vi "game_top_VI.vi"() -> ()   [LabVIEW 2014]
uses:
  <vilib>/Utility/miscctls.llb/LVPositionTypeDef.ctl
panel:
  in  "Stage Effects:":T1={"bar description"="ball will  speed up when pass aera: ", "brick discription"="ball will teleport \nand change speed: ", "y speed up"="◆□◆□◆□", "In : "=16711680, "Out : "=16711680, "x speed up"="■\n△\n■\n△\n△"}
  in  "leave":bool
  in  "Note":string="Score is calculated by :\n1. number of bricks breaked\n2. clear time of each level"
  in  "into pos 2":T2={"Left"=288, "Top"=-12}
  in  "into Pos":T2={"Left"=623, "Top"=-12}
  in  "OK Button":bool
  in  "Introoductions :":T3={"Bar : "=100, "bar description"="Move bar with key: \n  △    ■    ◆    □", "brick discription"="Use the ball to\nbreak the bricks", "Brick : "=0, "Ball : "=TRUE} {"Bar :" scale=0.0..100.0}
  in  "title":string="Brick Breaking Game"
  out "Top Ten High Score":T4(array[cluster])=[{"Placing"=1.0, "Name"="", "Score"=0.0, "Date"=""}, {"Placing"=2.0, "Name"="", "Score"=0.0, "Date"=""}, {"Placing"=3.0, "Name"="", "Score"=0.0, "Date"=""}, {"Placing"=4.0, "Name"="", "Score"=0.0, "Date"=""}, {"Placing"=5.0, "Name"="", "Score"=0.0, "Date"=""}, {"Placing"=6.0, "Name"="", "Score"=0.0, "Date"=""}, {"Placing"=7.0, "Name"="", "Score"=0.0, "Date"=""}, {"Placing"=8.0, "Name"="", "Score"=0.0, "Date"=""}, {"Placing"=9.0, "Name"="", "Score"=0.0, "Date"=""}, {"Placing"=10.0, "Name"="", "Score"=0.0, "Date"=""}]
  in  "Your Score":i32
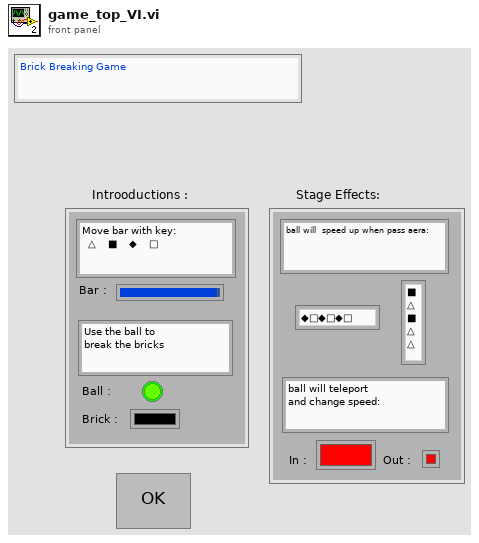
[diagram p1: front panel]
types:
  T1 = cluster{"bar description":string, "brick discription":string, "y speed up":string, "In : ":u32, "Out : ":u32, "x speed up":string}
  T2 = typedef "LVPositionTypeDef.ctl" = cluster{"Left":i32, "Top":i32}
  T3 = cluster{"Bar : ":u8, "bar description":string, "brick discription":string, "Brick : ":u32, "Ball : ":bool}
  T4 = cluster{"Placing":dbl, "Name":string, "Score":dbl, "Date":string}[]
  T5 = enum8{"Enabled", "Disabled", "Disabled and Grayed Out"}
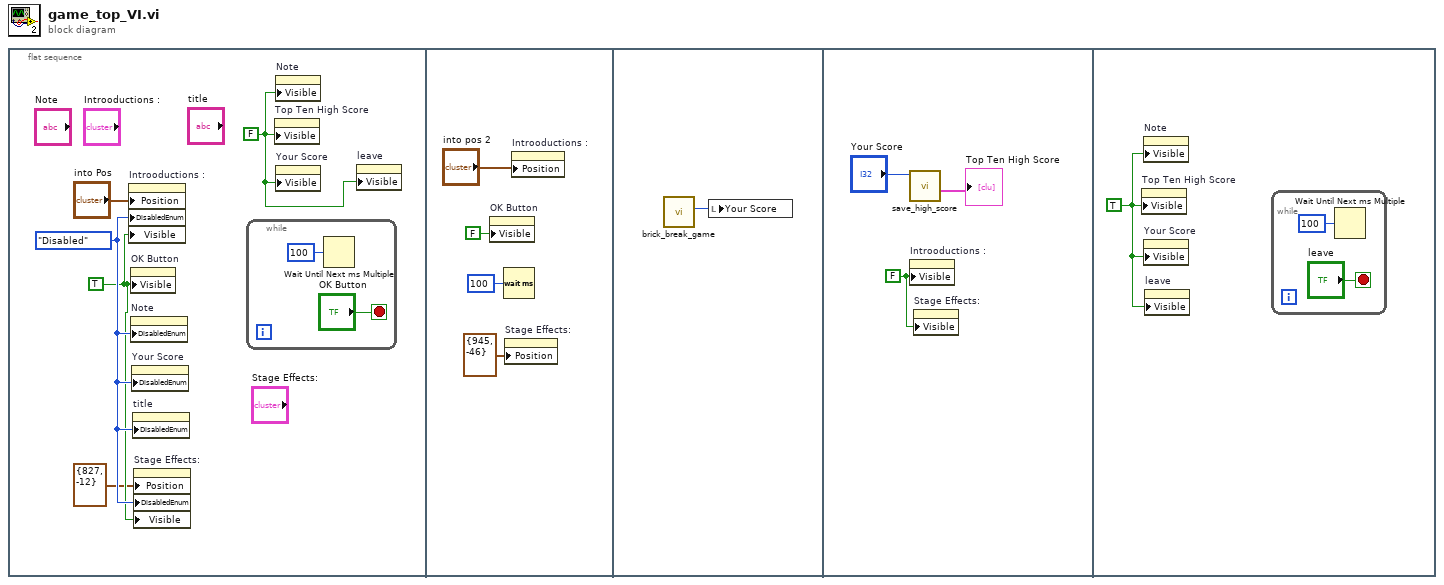
[diagram p0: block diagram]
diagram:
  n1 = flat-sequence {
    frame #0 {
      w4 = T5."Disabled" ("Disabled")
      w3 = TRUE ("Visible")
      w5 = FALSE
      n2 = property on="Introoductions :" class="Clust (strict)"("Position"="into Pos", "DisabledEnum"=w4, "Visible"=w3) -> ()  [unwired: 2 in, 2 out]
      n3 = property on="OK Button" class="Bool"("Visible"=w3) -> ()  [unwired: 2 in, 2 out]
      n4 = property on="Note" class="Str"("DisabledEnum"=w4) -> ()  [unwired: 2 in, 2 out]
      n5 = property on="Your Score" class="DigNum (strict)"("DisabledEnum"=w4) -> ()  [unwired: 2 in, 2 out]
      n6 = property on="title" class="Str"("DisabledEnum"=w4) -> ()  [unwired: 2 in, 2 out]
      n7 = property on="Stage Effects:" class="Clust (strict)"("Position"=T2 {"Left"=827, "Top"=-12}, "DisabledEnum"=w4, "Visible"=w3) -> ()  [unwired: 2 in, 2 out]
      n8 = while {
        stop <- "OK Button" stop-if-true
        n9 = Wait Until Next ms Multiple(millisecond multiple=u32 100 ("milliseconds to wait")) -> ()  [unwired: 1 out]
      }
      n10 = property on="Top Ten High Score" class="Arr (strict)"("Visible"=w5) -> ()  [unwired: 2 in, 2 out]
      n11 = property on="Note" class="Str"("Visible"=w5) -> ()  [unwired: 2 in, 2 out]
      n12 = property on="Your Score" class="DigNum (strict)"("Visible"=w5) -> ()  [unwired: 2 in, 2 out]
      n13 = property on="leave" class="Bool"("Visible"=w5) -> ()  [unwired: 2 in, 2 out]
    }
    frame #1 {
      n14 = property on="OK Button" class="Bool"("Visible"=FALSE) -> ()  [unwired: 2 in, 2 out]
      n15 = Wait (ms)(milliseconds to wait=u32 100) -> ()  [unwired: 1 out]
      n16 = property on="Stage Effects:" class="Clust (strict)"("Position"=T2 {"Left"=945, "Top"=-46}) -> ()  [unwired: 2 in, 2 out]
      n17 = property on="Introoductions :" class="Clust (strict)"("Position"="into pos 2") -> ()  [unwired: 2 in, 2 out]
    }
    frame #2 {
      n18 = call "brick_break_game.vi"() -> ("Score"=w12:i32)  [unwired: 11 in]
      n19 = local write "Your Score"(w12) -> ()
    }
    frame #3 {
      w13 = FALSE ("Visible")
      n20 = call "save_high_score.vi"("Your Score"="Your Score") -> ("Top Ten High Score 2"=→"Top Ten High Score":T4)  [unwired: 10 in]
      n21 = property on="Introoductions :" class="Clust (strict)"("Visible"=w13) -> ()  [unwired: 2 in, 2 out]
      n22 = property on="Stage Effects:" class="Clust (strict)"("Visible"=w13) -> ()  [unwired: 2 in, 2 out]
    }
    frame #4 {
      w16 = TRUE
      n23 = property on="Top Ten High Score" class="Arr (strict)"("Visible"=w16) -> ()  [unwired: 2 in, 2 out]
      n24 = property on="Note" class="Str"("Visible"=w16) -> ()  [unwired: 2 in, 2 out]
      n25 = property on="Your Score" class="DigNum (strict)"("Visible"=w16) -> ()  [unwired: 2 in, 2 out]
      n26 = property on="leave" class="Bool"("Visible"=w16) -> ()  [unwired: 2 in, 2 out]
      n27 = while {
        stop <- "leave" stop-if-true
        n28 = Wait Until Next ms Multiple(millisecond multiple=u32 100 ("milliseconds to wait")) -> ()  [unwired: 1 out]
      }
    }
  }
